vi "1D Fourier Interpolation.vi"() -> ()   [LabVIEW 2023]
doc: "This example shows the operation of the 1D Fourier interpolation VI by transforming an array to the frequency domain, and then transforming it back to the time domain to form the output interpolated array. The different data generation parameters allow adding different frequencies, changing sampling and # of samples information, adding noise and offset. The interpolation parameters allow determination of the number of points to be interpolated between each given Y points."
uses:
  <vilib>/gmath/NI_Gmath.lvlib
  <vilib>/measure/NI_MABase.lvlib
panel:
  in  "Stop":bool
  in  "Noise (rms)":dbl(knob) scale=0.0..0.1
  in  "Offset":dbl(slide) scale=-2.0..2.0
  in  "Sampling info":cluster{"Fs":dbl, "#s":dbl}={"Fs"=1002.0, "#s"=50.0}
  in  "Tone":T1(array[cluster])=[{"frequency"=100.0, "amplitude"=1.0, "phase"=0.0}, {"frequency"=20.0, "amplitude"=1.0, "phase"=0.0}]
  in  "Interpolation factor (n)":i32(slide)=2 scale=0.0..10.0
  out "Interpolation Graph":waveform(dbl)[](graph)
  # "Overview: Demonstrates the use of the Interpolate 1D Fourier VI.\nRequirements: LabVIEW Full Development System\nInstructions:\n1. Run the VI.\n2. Modify the Tone and Interpolation factor parameters and observe the effect on the Interpolation Graph.\n3. Click Stop to stop the VI."
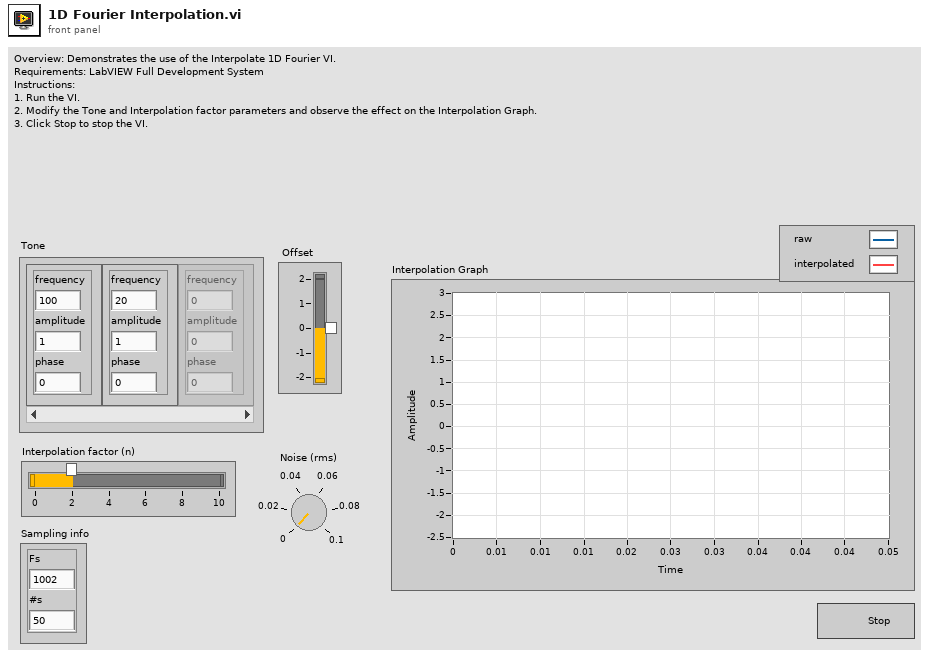
[diagram p1: front panel]
types:
  T1 = cluster{"frequency":dbl, "amplitude":dbl, "phase":dbl}[]
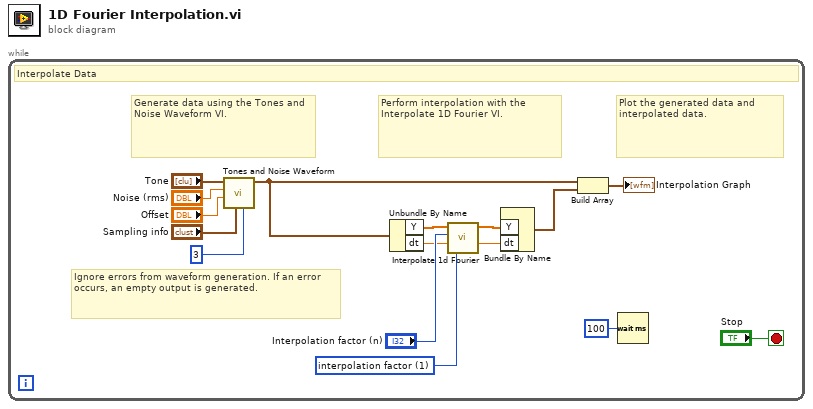
[diagram p0: block diagram]
diagram:
  n1 = while {
    stop <- "Stop" stop-if-true
    w1 = u16 1 items=["interpolation size", "interpolation factor"] ("type")
    # "Ignore errors from waveform generation. If an error occurs, an empty output is generated."
    # "Generate data using the Tones and Noise Waveform VI."
    # "Plot the generated data and interpolated data."
    # "Perform interpolation with the Interpolate 1D Fourier VI."
    # "Interpolate Data"
    n2 = call <vilib>:"Tones and Noise Waveform.vi"("seed"=3, "sampling info"="Sampling info", "offset"="Offset", "noise (rms)"="Noise (rms)", "tones"="Tone") -> ("signal out"=w5:waveform(dbl))  [unwired: 5 in, 1 out]
    n3 = Unbundle By Name(w5) -> ("Y"=w4:dbl[], "dt"=w7:dbl)
    n4 = call <vilib>:"Interpolate 1d Fourier.vi"("type"=w1, "dt in"=w7, "n"="Interpolation factor (n)", "X"=w4) -> ("dt out"=w6:dbl, "Y"=w11:dbl[])  [unwired: 4 in, 2 out]
    n5 = Bundle By Name("Y"=w11, "dt"=w6) -> (w15:waveform(dbl))  [unwired: 1 in]
    n6 = Build Array(w5, w15) -> (→"Interpolation Graph":waveform(dbl)[])
    n7 = Wait (ms)(milliseconds to wait=u32 100 ("millisecond multiple")) -> ()  [unwired: 1 out]
  }
